vi "sk-watertunnel-control-9-10-16.vi"() -> ()   [LabVIEW 2012]
uses:
  <vilib>/Utility/error.llb/DialogType.ctl
  <vilib>/DAQmx/write.llb/DAQmx Write (Digital 1D Wfm NChan NSamp).vi
  <vilib>/DAQmx/write.llb/DAQmx Write (Analog Wfm 1Chan NSamp).vi
  <vilib>/DAQmx/write.llb/DAQmx Write (Analog DBL 1Chan 1Samp).vi
  <vilib>/DAQmx/write.llb/DAQmx Write (Digital 1D Bool 1Chan 1Samp).vi
  <vilib>/Instr/_visa.llb/VISA Configure Serial Port (Instr).vi
  <vilib>/DAQmx/create/channels.llb/DAQmx Create Channel (AO-Voltage-Basic).vi
  <vilib>/DAQmx/create/channels.llb/DAQmx Create Channel (DO-Digital Output).vi
  <vilib>/Waveform/DWDTOps.llb/DWDT Analog to Digital.vi
  <vilib>/DAQmx/configure/timing.llb/DAQmx Timing (Sample Clock).vi
  <vilib>/DAQmx/create/channels.llb/DAQmx Create Channel (CO-Pulse Generation-Time).vi
  <vilib>/DAQmx/configure/trigger.llb/DAQmx Start Trigger (Digital Edge).vi
  <vilib>/DAQmx/miscellaneous.llb/DAQmx Fill In Error Info.vi
  <vilib>/Waveform/DWDTOps.llb/DWDT Uncompress Digital.vi
  <vilib>/measure/NI_MABase.lvlib
panel:
  in  "RECORD":bool
  in  "select path":path=path "D:/skramel/labview/hex-9-6-2016-2-15-1-01.txt"
  in  "VISA resource name 5":refnum<visa-resource-name>="COM105"
  in  "VISA resource name 4":refnum<visa-resource-name>="COM104"
  in  "VISA resource name 3":refnum<visa-resource-name>="COM103"
  in  "VISA resource name 2":refnum<visa-resource-name>="COM102"
  in  "Select Program":i32(ring)=1 items=["Manual Control", "Read from .txt file"]
  in  "stop":bool
  out "Current Command in .txt file - board 1":string="relay writeall 30\r"
  out "Current Command in .txt file - board 2":string="relay writeall 00\r"
  out "Current Command in .txt file - board 3":string="relay writeall 23\r"
  out "Current Command in .txt file - board 4":string="relay writeall 04\r"
  out "Current Command in .txt file - board 5":string="relay writeall 44\r"
  in  "Serial write":bool=TRUE
  in  "stop 2":bool
  in  "R 1":bool=TRUE
  in  "R 2":bool=TRUE
  in  "R 3":bool=TRUE
  in  "R 4":bool=TRUE
  in  "R 5":bool=TRUE
  in  "R 6":bool=TRUE
  in  "R 9":bool=TRUE
  in  "R 10":bool=TRUE
  in  "R 11":bool=TRUE
  in  "R 12":bool=TRUE
  in  "R 13":bool=TRUE
  in  "R 14":bool=TRUE
  in  "R 15":bool=TRUE
  in  "R 16":bool=TRUE
  in  "R 7":bool=TRUE
  in  "R 8":bool=TRUE
  in  "R 17":bool=TRUE
  in  "R 18":bool=TRUE
  in  "R 19":bool=TRUE
  in  "R 20":bool=TRUE
  in  "R 21":bool=TRUE
  in  "R 22":bool=TRUE
  in  "R 31":bool=TRUE
  in  "R 32":bool=TRUE
  in  "R 23":bool=TRUE
  in  "R 24":bool=TRUE
  in  "R 25":bool=TRUE
  in  "R 26":bool=TRUE
  in  "R 27":bool=TRUE
  in  "R 28":bool=TRUE
  in  "R 29":bool=TRUE
  in  "R 30":bool=TRUE
  out "Current Command (manual control) - board 1":string="relay writeall 00\r"
  in  "R 33":bool=TRUE
  in  "R 34":bool=TRUE
  in  "R 35":bool=TRUE
  in  "R 36":bool=TRUE
  in  "R 37":bool=TRUE
  in  "R 38":bool=TRUE
  in  "R 39":bool=TRUE
  in  "R 40":bool=TRUE
  out "Current Command (manual control) - board 2":string="relay writeall 00\r"
  out "board 5":string="00"
  in  "Manual Override - turn all relays off":bool=TRUE
  out "board 1":string="00"
  out "board 2":string="00"
  out "board 3":string="00"
  out "board 4":string="00"
  out "Current Command (manual control) - board 3":string="relay writeall 00\r"
  out "Current Command (manual control) - board 4":string="relay writeall 00\r"
  out "Current Command (manual control) - board 5":string="relay writeall 00\r"
  in  "Serial write update rate (ms)":u32=100
  in  "End write with termination character?":bool=TRUE
  in  "Input buffer size":u32=4096
  in  "termination char\n(0xA = '\\n' = LF\n0xD = '\\r' = CR)":u8=13 format="%.0x"
  in  "End read on termination character?":bool=TRUE
  in  "timeout (ms)":u32=10000
  in  "stop bits":u16(ring)=10 items=["1.0"=10, "1.5"=15, "2.0"=20]
  in  "parity":u16(ring) items=["None", "Odd", "Even", "Mark", "Space"]
  in  "data bits":u16=8 min=5 max=8 step=1
  in  "VISA resource name 1":refnum<visa-resource-name>="COM101"
  in  "baud rate":u32=9600
  in  "Physical Channel":tag="Dev1/ao1" caption="Analog Output (LED Trigger - Black Wire)"
  in  "duty cycle (%)":dbl=10.0 format="%0.2f"
  in  "phase":dbl format="%.2p"
  in  "amplitude":dbl=10.0 format="%0.2p"
  in  "frequency":dbl=450.0 format="%0.2p"
  in  "STOP":bool
  in  "sampling info":cluster{"Fs":dbl, "#s":dbl}={"Fs"=450000.0, "#s"=450000.0} {"Fs" format="%.2p"}
  in  "duty cycle (%)":dbl=50.0 format="%0.2f"
  in  "phase":dbl format="%.2p"
  in  "amplitude":dbl=1.0 format="%0.2p"
  in  "frequency":dbl=450.0 format="%0.2p"
  in  "Sample Clock Rate":dbl=450000.0 format="%.2f"
  in  "Digital Output (Camera Trigger)":tag="Dev1/port0/line0:1" caption="Physical Channels"
  in  "On / Off":bool=TRUE
  in  "Voltage Output":dbl(slide)=10.0 min=0.0 max=10.0 scale=0.0..10.0 scale format="%.3f"
  in  "Maximum Value":dbl=10.0 format="%0.2f"
  in  "Minimum Value":dbl format="%0.2f"
  in  "Physical Channel":tag="Dev1/ao0" caption="Analog Output (LED Intensity - Grey Wire)"
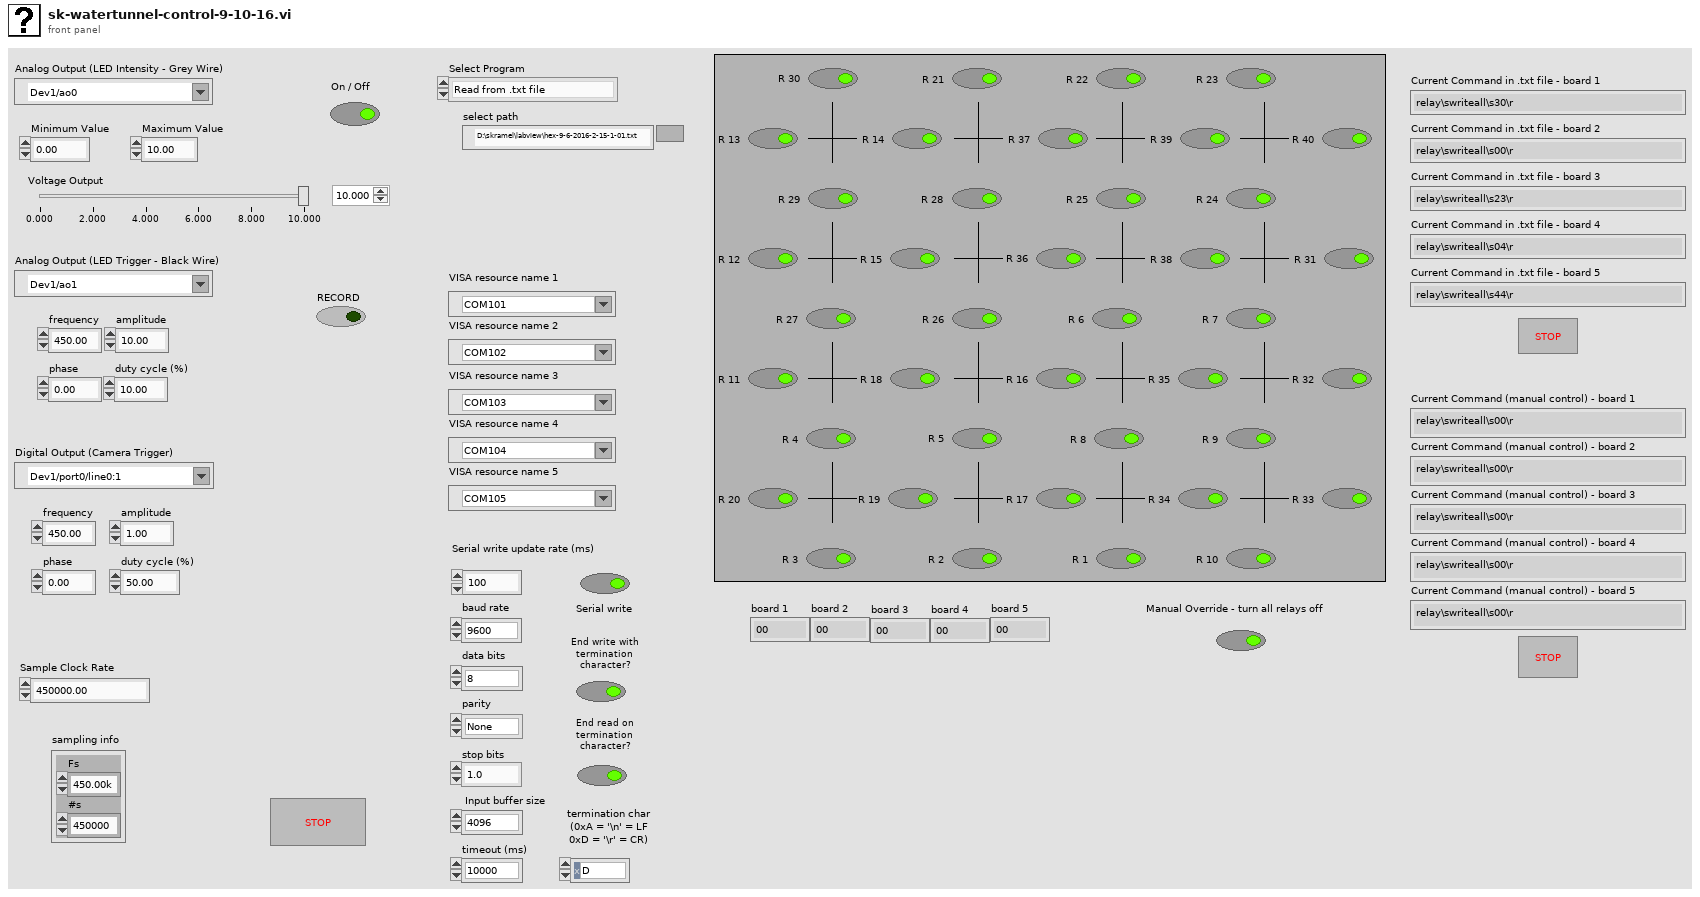
[diagram p1: front panel]
types:
  T1 = enum16{"open", "replace", "create", "open or create", "replace or create", "replace or create with confirmation"}
  T2 = typedef "DialogType.ctl" = u16
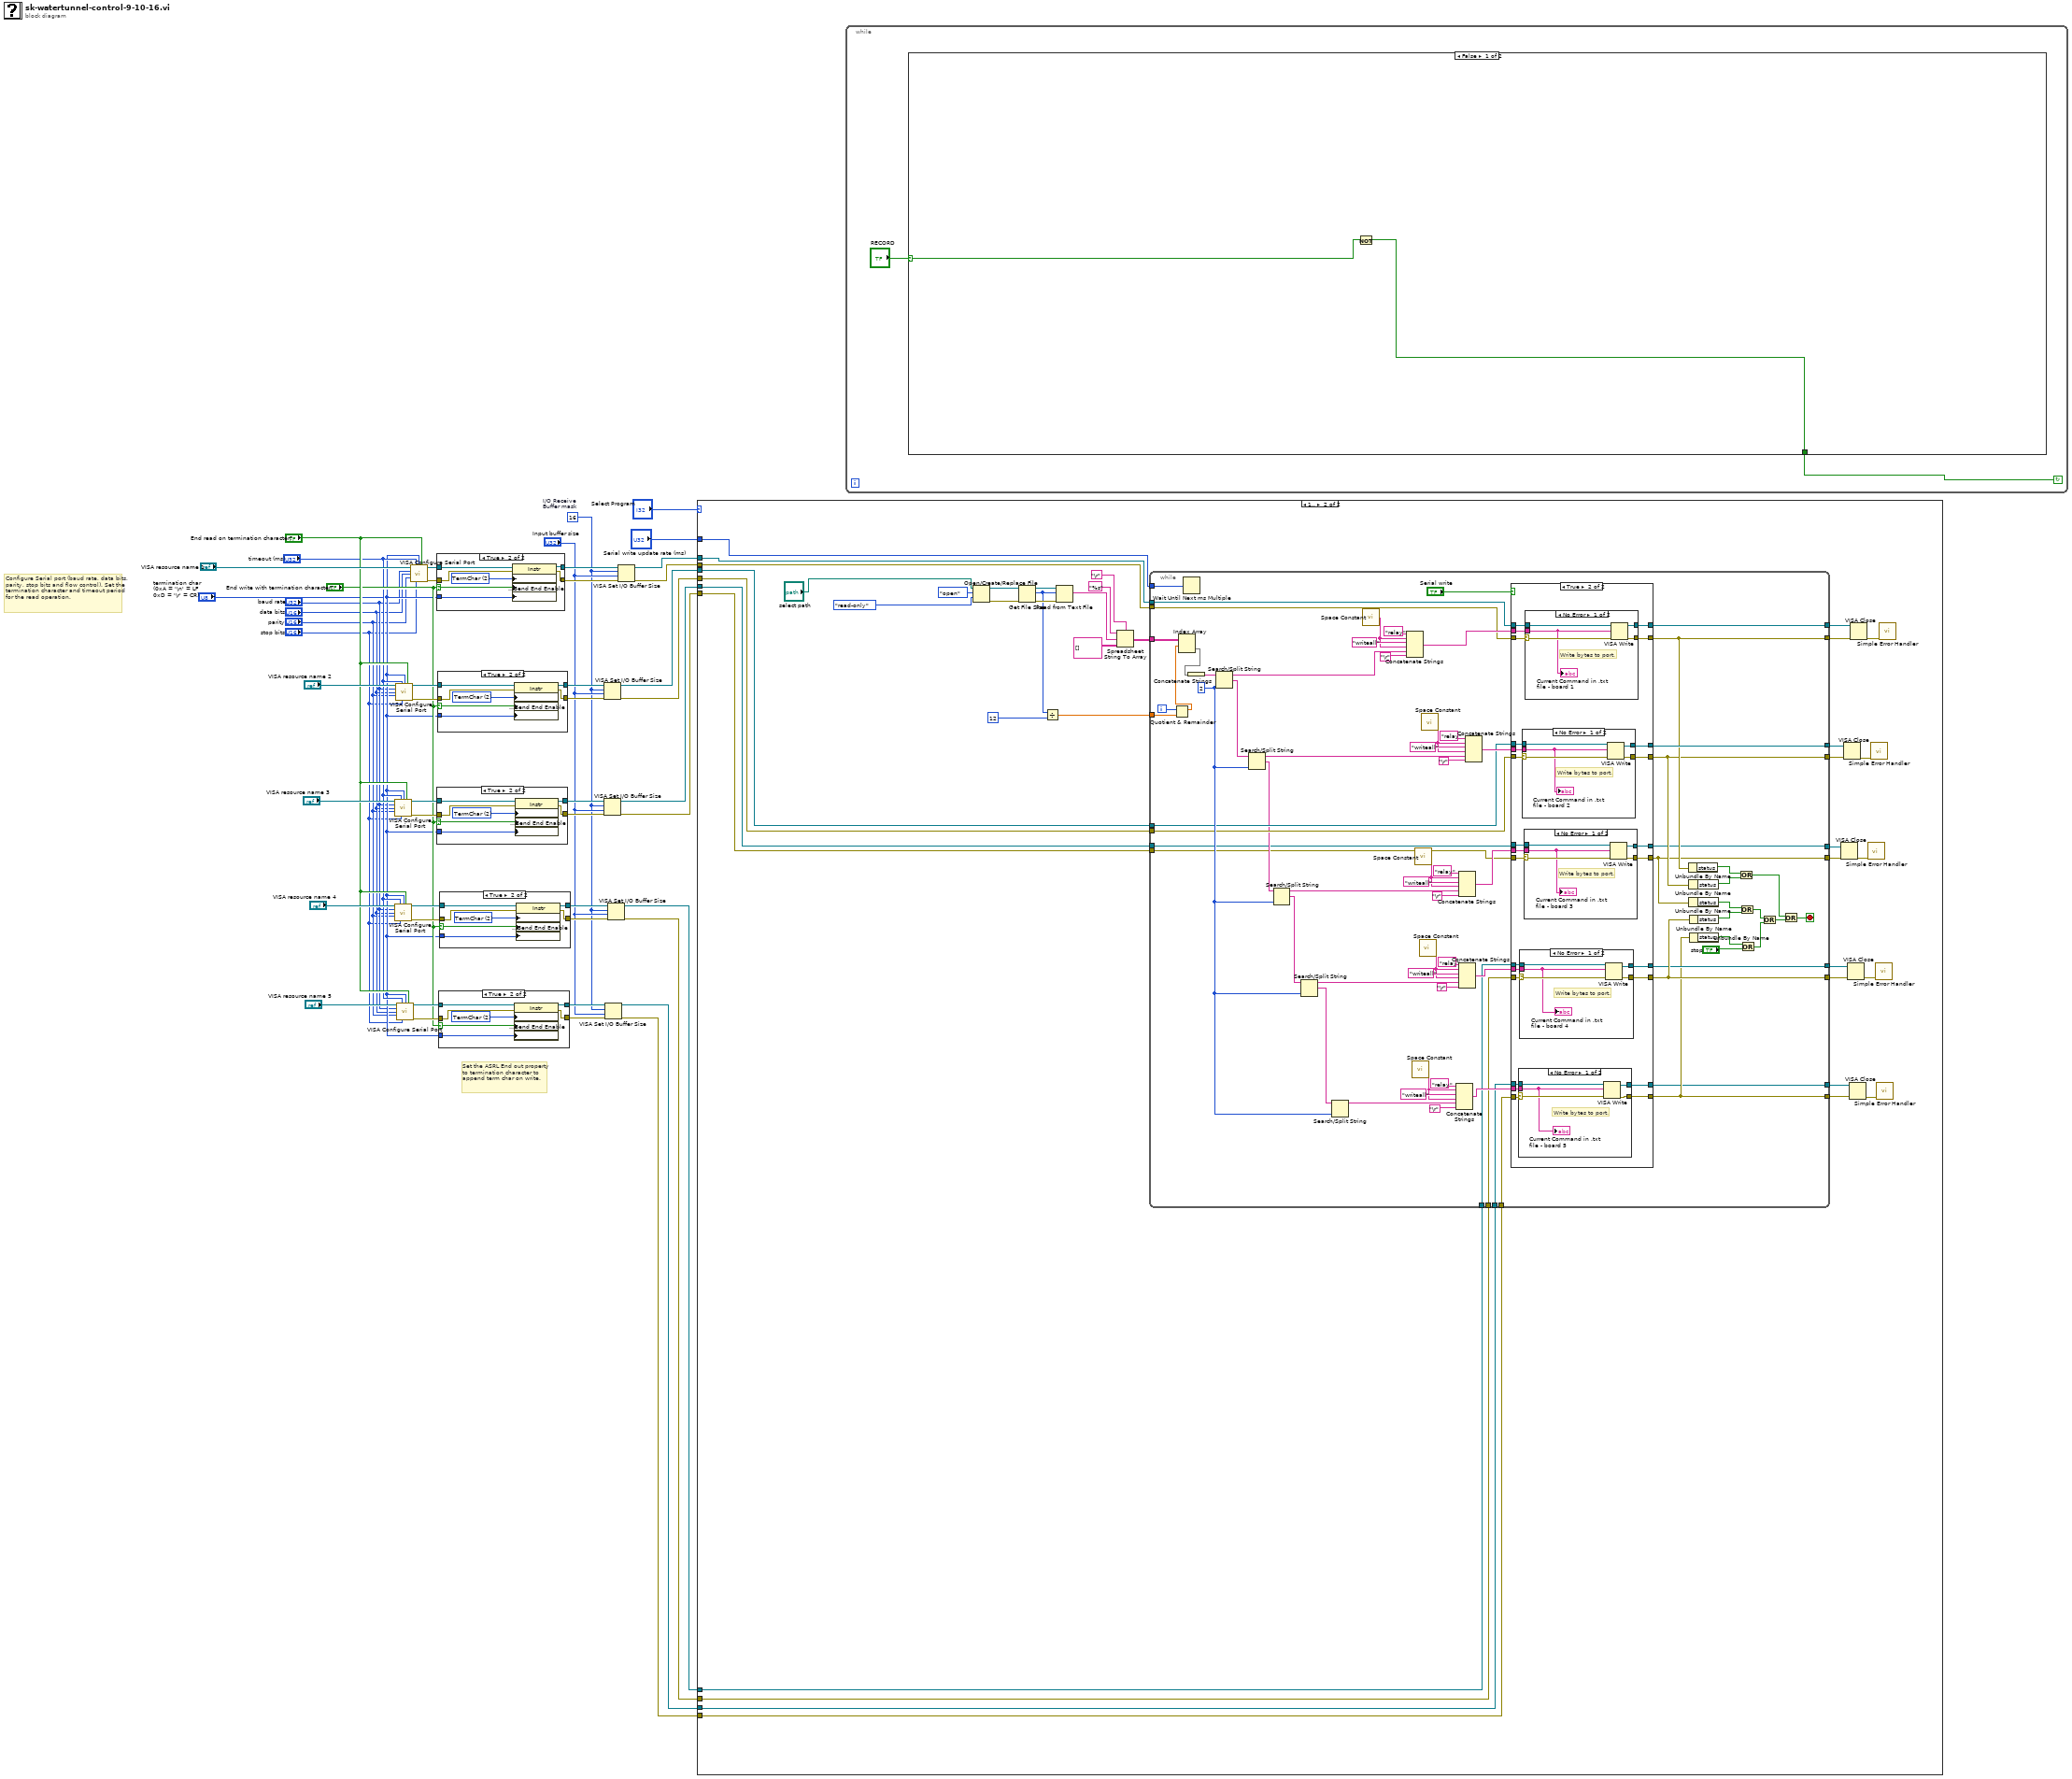
[diagram p0: block diagram]
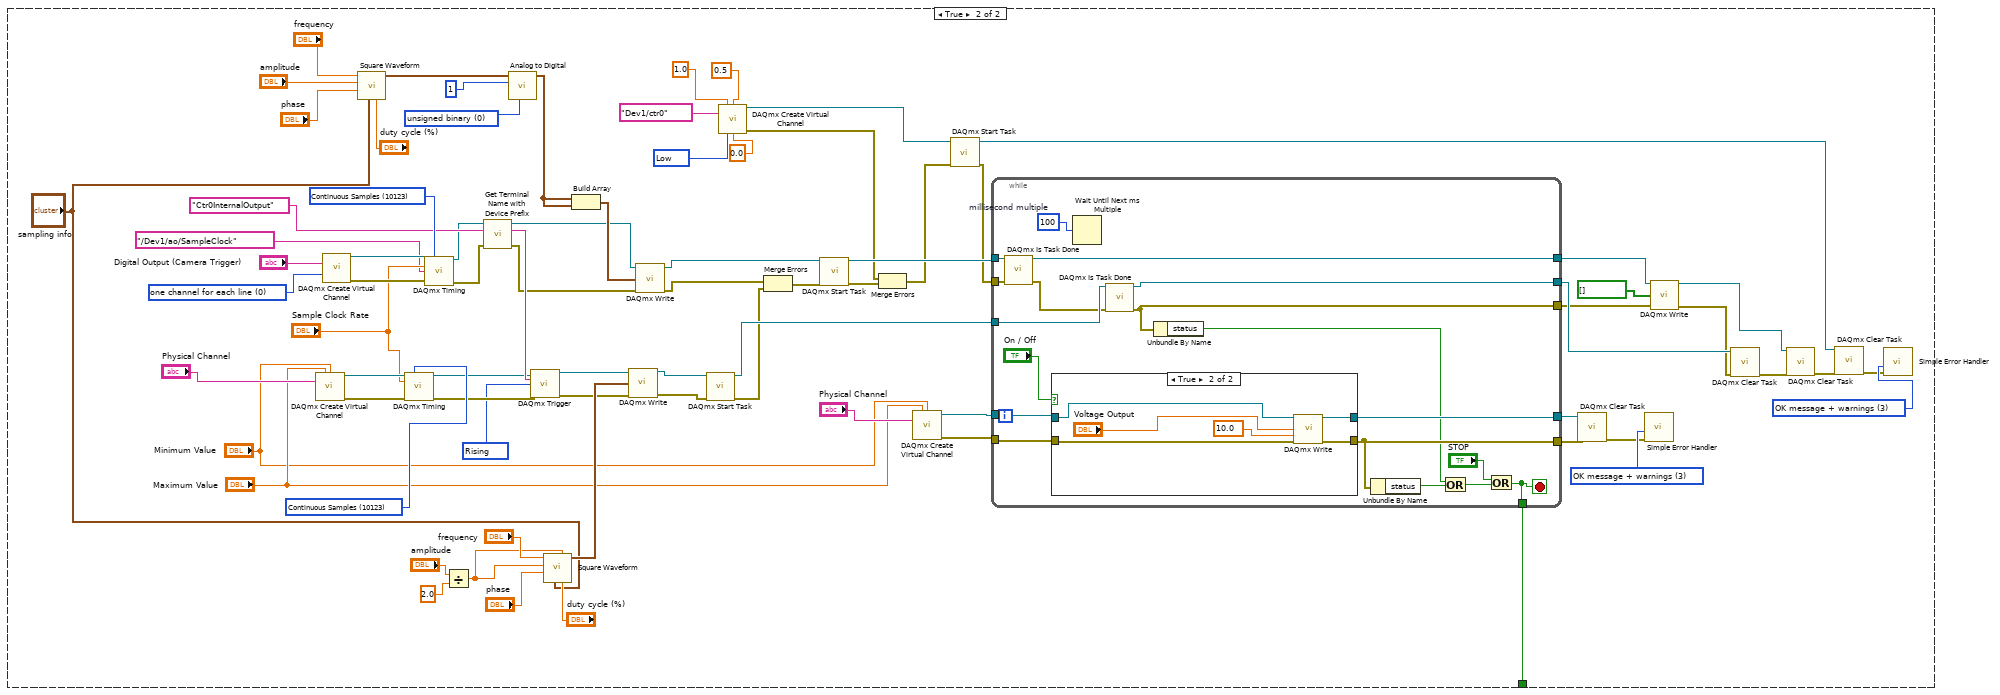
[diagram p2: hidden frame]
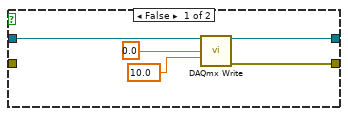
[diagram p3: hidden frame]
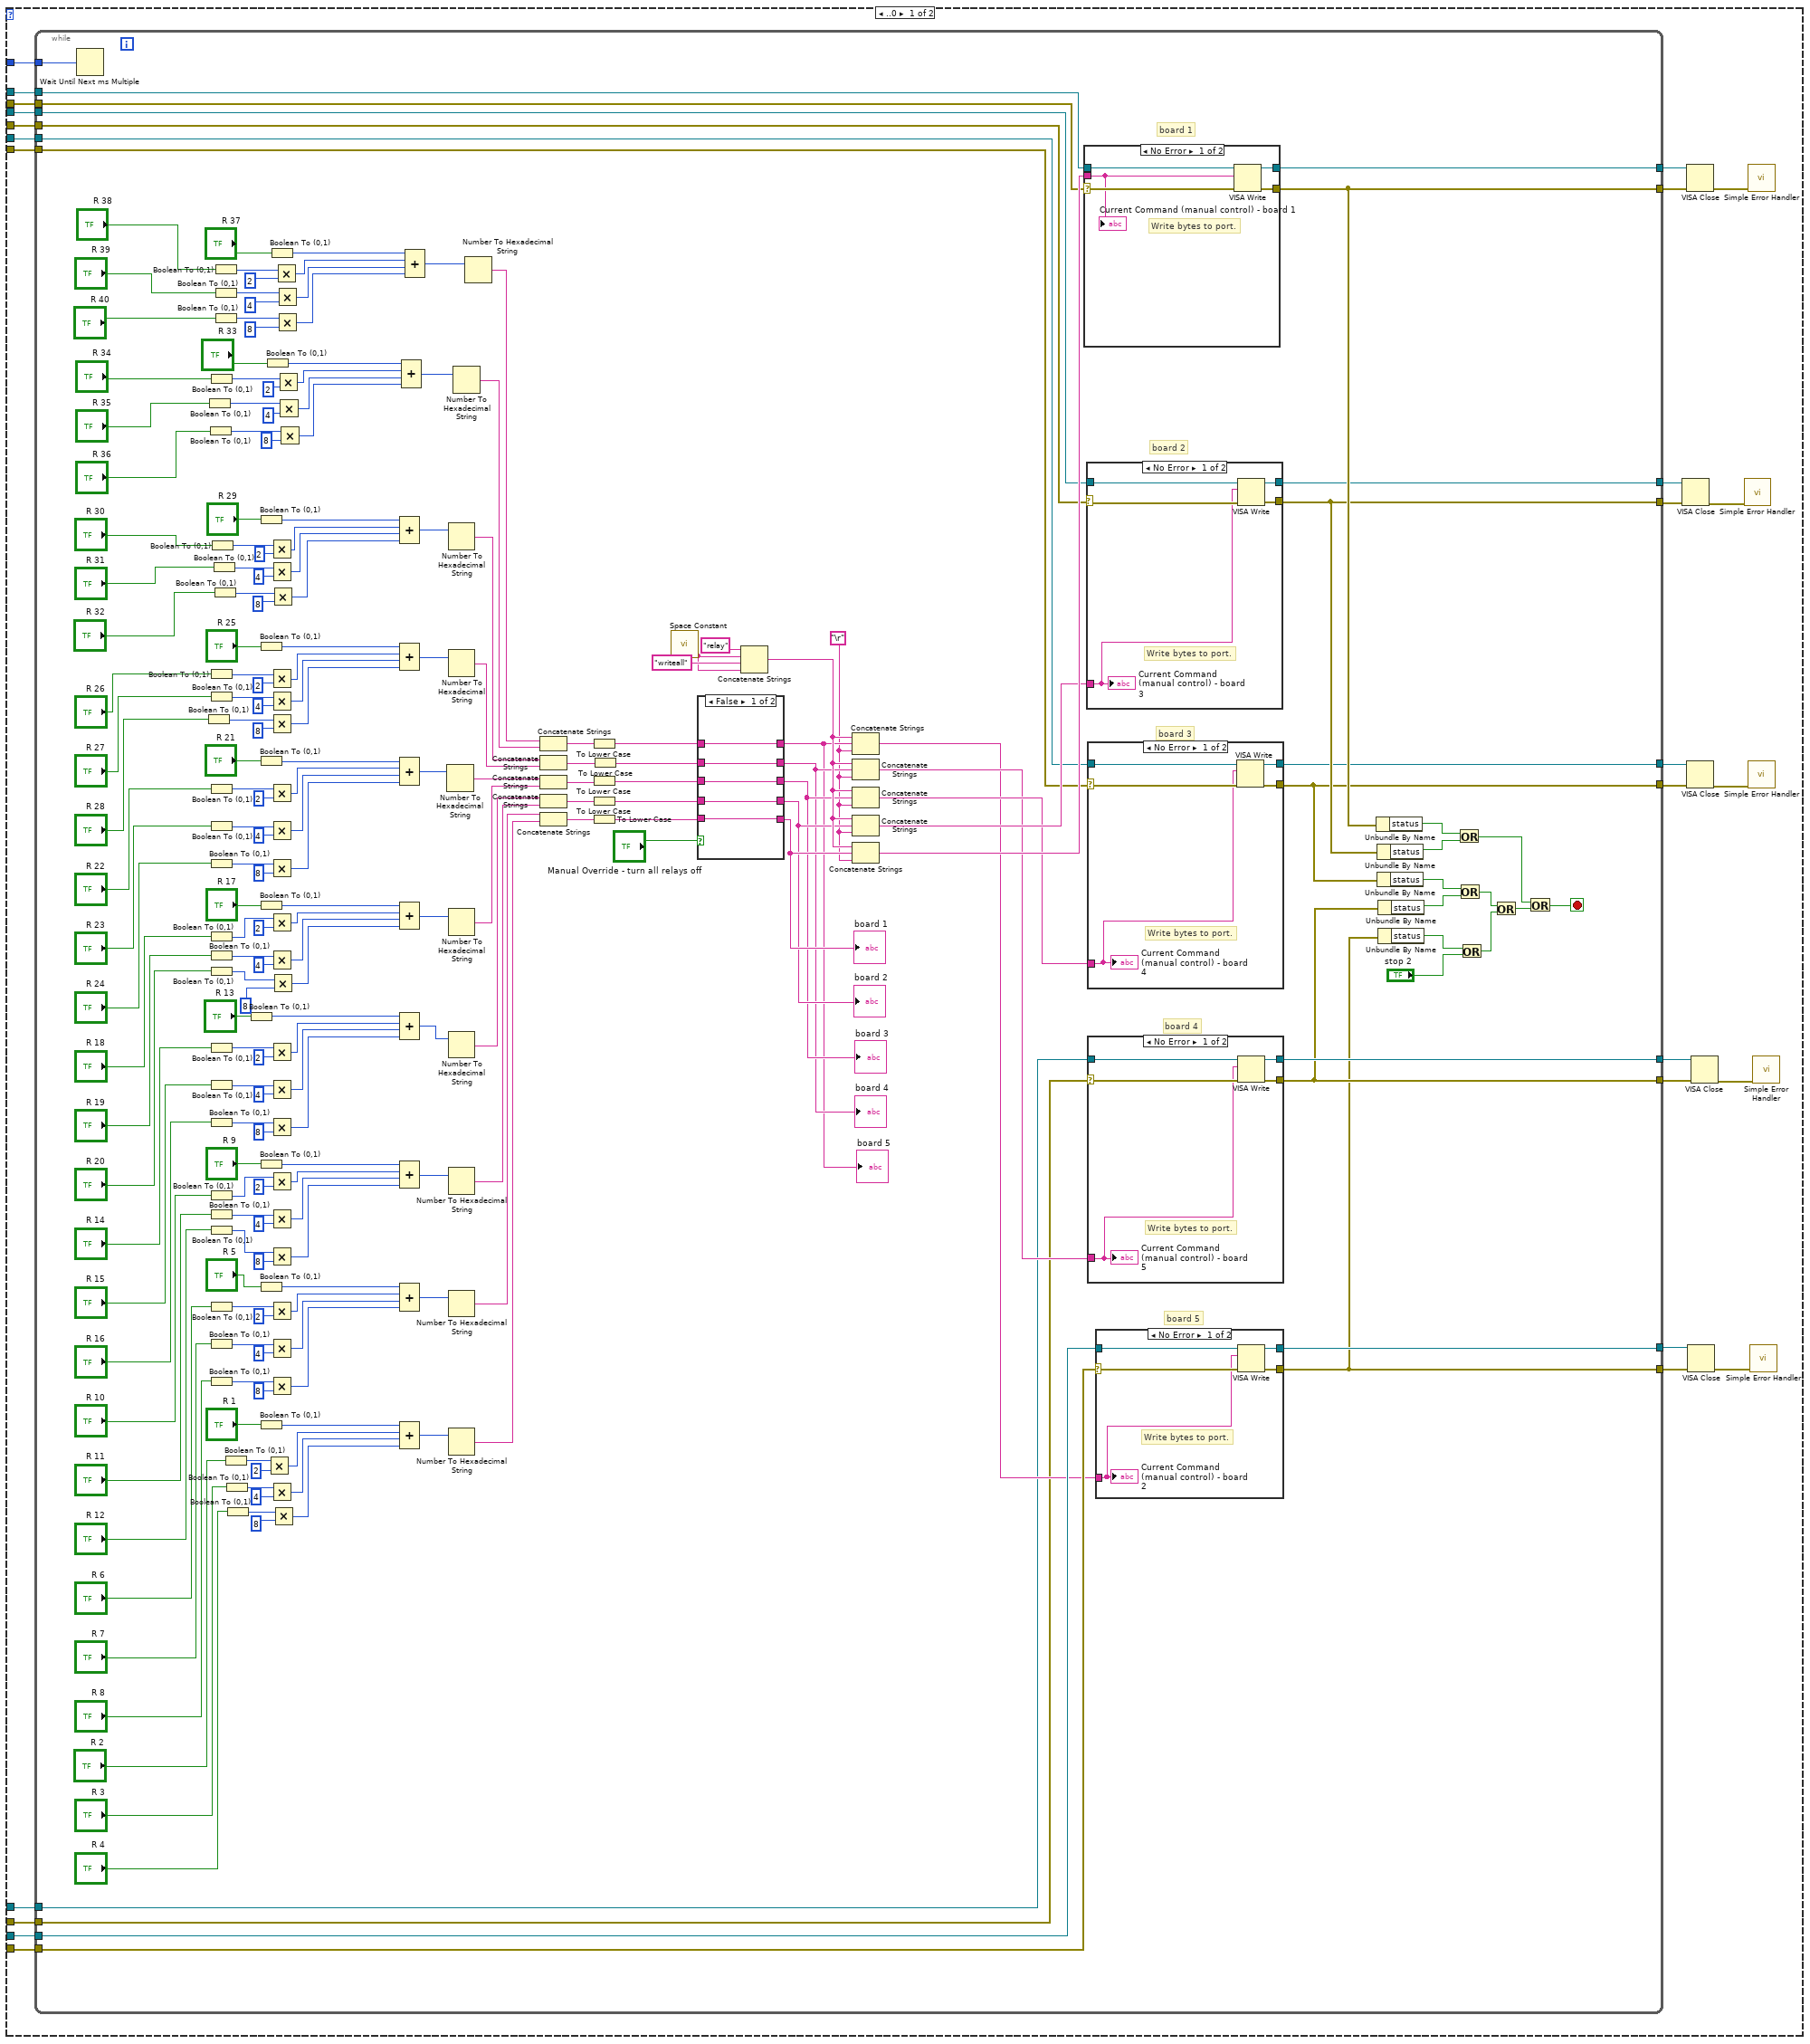
[diagram p8: hidden frame]
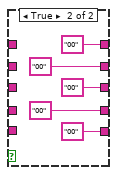
[diagram p12: hidden frame]
diagram:
  w1 = u16 16  # I/O Receive Buffer mask
  # "Set the ASRL End out property to termination character to append term char on write."
  # "Configure Serial port (baud rate, data bits, parity, stop bits and flow control). Set the termination character and timeout period for the read operation."
  n1 = call-poly "VISA Configure Serial Port"("VISA resource name"="VISA resource name 4", "timeout (10sec)"="timeout (ms)", "termination char\n(0xA = '\\n' = LF)"="termination char\n(0xA = '\\n' = LF\n0xD = '\\r' = CR)", "Enable Termination\nChar (T)"="End read on termination character?", "baud rate (9600)"="baud rate", "data bits (8)"="data bits", "parity (0:none)"="parity", "stop bits (10: 1 bit)"="stop bits") -> ("VISA resource name out"=w23:refnum<visa-resource-name>, "error out"=w26:errorcluster)  [unwired: 2 in, 4 out]
  n2 = call-poly "VISA Configure Serial Port"("VISA resource name"="VISA resource name 3", "timeout (10sec)"="timeout (ms)", "termination char\n(0xA = '\\n' = LF)"="termination char\n(0xA = '\\n' = LF\n0xD = '\\r' = CR)", "Enable Termination\nChar (T)"="End read on termination character?", "baud rate (9600)"="baud rate", "data bits (8)"="data bits", "parity (0:none)"="parity", "stop bits (10: 1 bit)"="stop bits") -> ("VISA resource name out"=w28:refnum<visa-resource-name>, "error out"=w31:errorcluster)  [unwired: 2 in, 4 out]
  n3 = call-poly "VISA Configure Serial Port"("VISA resource name"="VISA resource name 2", "timeout (10sec)"="timeout (ms)", "termination char\n(0xA = '\\n' = LF)"="termination char\n(0xA = '\\n' = LF\n0xD = '\\r' = CR)", "Enable Termination\nChar (T)"="End read on termination character?", "baud rate (9600)"="baud rate", "data bits (8)"="data bits", "parity (0:none)"="parity", "stop bits (10: 1 bit)"="stop bits") -> ("VISA resource name out"=w35:refnum<visa-resource-name>, "error out"=w38:errorcluster)  [unwired: 2 in, 4 out]
  n4 = call-poly "VISA Configure Serial Port"("VISA resource name"="VISA resource name 5", "timeout (10sec)"="timeout (ms)", "termination char\n(0xA = '\\n' = LF)"="termination char\n(0xA = '\\n' = LF\n0xD = '\\r' = CR)", "Enable Termination\nChar (T)"="End read on termination character?", "baud rate (9600)"="baud rate", "data bits (8)"="data bits", "parity (0:none)"="parity", "stop bits (10: 1 bit)"="stop bits") -> ("VISA resource name out"=w18:refnum<visa-resource-name>, "error out"=w21:errorcluster)  [unwired: 2 in, 4 out]
  n5 = call-poly "VISA Configure Serial Port"("VISA resource name"="VISA resource name 1", "timeout (10sec)"="timeout (ms)", "termination char\n(0xA = '\\n' = LF)"="termination char\n(0xA = '\\n' = LF\n0xD = '\\r' = CR)", "Enable Termination\nChar (T)"="End read on termination character?", "baud rate (9600)"="baud rate", "data bits (8)"="data bits", "parity (0:none)"="parity", "stop bits (10: 1 bit)"="stop bits") -> ("VISA resource name out"=w43:refnum<visa-resource-name>, "error out"=w46:errorcluster)  [unwired: 2 in, 4 out]
  n6 = case shown="True" "End write with termination character?" {
    selector: "End write with termination character?" -> [_ w51]
    tunnel: w43 -> [w48 w56]
    tunnel: w46 -> [w49 w55]
    tunnel: [w48 w54] -> w44
    tunnel: [w49 w50] -> w45
    tunnel: "termination char\n(0xA = '\\n' = LF\n0xD = '\\r' = CR)" -> [_ w52]
    frame False {
    }
    frame True {
      w53 = u16 2 items=["None", "LastBit", "TermChar", "Break"] ("Serial Settings:Serial End Mode for Writes")
      n7 = property class="Instr"(reference=w56, error in=w55, "Serial Settings:End Mode for Writes"=w53, "Message Based Settings:Send End Enable"=w51, "Message Based Settings:Termination Character"=w52) -> (reference out=w54:refnum<visa-resource-name>, error out=w50:errorcluster)
    }
  }
  n8 = case shown="True" "End write with termination character?" {
    selector: "End write with termination character?" -> [_ w60]
    tunnel: w28 -> [w57 w65]
    tunnel: w31 -> [w58 w64]
    tunnel: [w57 w63] -> w29
    tunnel: [w58 w62] -> w30
    tunnel: "termination char\n(0xA = '\\n' = LF\n0xD = '\\r' = CR)" -> [_ w59]
    frame False {
    }
    frame True {
      w61 = u16 2 items=["None", "LastBit", "TermChar", "Break"] ("Serial Settings:Serial End Mode for Writes")
      n9 = property class="Instr"(reference=w65, error in=w64, "Serial Settings:End Mode for Writes"=w61, "Message Based Settings:Send End Enable"=w60, "Message Based Settings:Termination Character"=w59) -> (reference out=w63:refnum<visa-resource-name>, error out=w62:errorcluster)
    }
  }
  n10 = case shown="True" "End write with termination character?" {
    selector: "End write with termination character?" -> [_ w69]
    tunnel: w35 -> [w66 w74]
    tunnel: w38 -> [w67 w73]
    tunnel: [w66 w72] -> w36
    tunnel: [w67 w71] -> w37
    tunnel: "termination char\n(0xA = '\\n' = LF\n0xD = '\\r' = CR)" -> [_ w68]
    frame False {
    }
    frame True {
      w70 = u16 2 items=["None", "LastBit", "TermChar", "Break"] ("Serial Settings:Serial End Mode for Writes")
      n11 = property class="Instr"(reference=w74, error in=w73, "Serial Settings:End Mode for Writes"=w70, "Message Based Settings:Send End Enable"=w69, "Message Based Settings:Termination Character"=w68) -> (reference out=w72:refnum<visa-resource-name>, error out=w71:errorcluster)
    }
  }
  n12 = case shown="True" "End write with termination character?" {
    selector: "End write with termination character?" -> [_ w78]
    tunnel: w18 -> [w75 w83]
    tunnel: w21 -> [w76 w82]
    tunnel: [w75 w81] -> w19
    tunnel: [w76 w80] -> w20
    tunnel: "termination char\n(0xA = '\\n' = LF\n0xD = '\\r' = CR)" -> [_ w77]
    frame False {
    }
    frame True {
      w79 = u16 2 items=["None", "LastBit", "TermChar", "Break"] ("Serial Settings:Serial End Mode for Writes")
      n13 = property class="Instr"(reference=w83, error in=w82, "Serial Settings:End Mode for Writes"=w79, "Message Based Settings:Send End Enable"=w78, "Message Based Settings:Termination Character"=w77) -> (reference out=w81:refnum<visa-resource-name>, error out=w80:errorcluster)
    }
  }
  n14 = case shown="True" "End write with termination character?" {
    selector: "End write with termination character?" -> [_ w87]
    tunnel: w23 -> [w84 w92]
    tunnel: w26 -> [w85 w91]
    tunnel: [w84 w90] -> w24
    tunnel: [w85 w89] -> w25
    tunnel: "termination char\n(0xA = '\\n' = LF\n0xD = '\\r' = CR)" -> [_ w86]
    frame False {
    }
    frame True {
      w88 = u16 2 items=["None", "LastBit", "TermChar", "Break"] ("Serial Settings:Serial End Mode for Writes")
      n15 = property class="Instr"(reference=w92, error in=w91, "Serial Settings:End Mode for Writes"=w88, "Message Based Settings:Send End Enable"=w87, "Message Based Settings:Termination Character"=w86) -> (reference out=w90:refnum<visa-resource-name>, error out=w89:errorcluster)
    }
  }
  n16 = VISA Set I/O Buffer Size(VISA resource name=w29, mask (16)=w1, size (4096)="Input buffer size", error in (no error)=w30) -> (VISA resource name out=w8:refnum<visa-resource-name>, error out=w7:errorcluster)
  n17 = VISA Set I/O Buffer Size(VISA resource name=w36, mask (16)=w1, size (4096)="Input buffer size", error in (no error)=w37) -> (VISA resource name out=w34:refnum<visa-resource-name>, error out=w33:errorcluster)
  n18 = VISA Set I/O Buffer Size(VISA resource name=w19, mask (16)=w1, size (4096)="Input buffer size", error in (no error)=w20) -> (VISA resource name out=w5:refnum<visa-resource-name>, error out=w6:errorcluster)
  n19 = VISA Set I/O Buffer Size(VISA resource name=w24, mask (16)=w1, size (4096)="Input buffer size", error in (no error)=w25) -> (VISA resource name out=w3:refnum<visa-resource-name>, error out=w4:errorcluster)
  n20 = VISA Set I/O Buffer Size(VISA resource name=w44, mask (16)=w1, size (4096)="Input buffer size", error in (no error)=w45) -> (VISA resource name out=w42:refnum<visa-resource-name>, error out=w41:errorcluster)
  n21 = case shown="1.." "Select Program" {
    tunnel: w42 -> [w114 w410]
    tunnel: w41 -> [w110 w409]
    tunnel: "Serial write update rate (ms)" -> [w115 w408]
    tunnel: w34 -> [w109 w407]
    tunnel: w33 -> [w108 w406]
    tunnel: w8 -> [w107 w384]
    tunnel: w7 -> [w106 w383]
    tunnel: w6 -> [w105 w385]
    tunnel: w5 -> [w104 w386]
    tunnel: w4 -> [w103 w387]
    tunnel: w3 -> [w102 w388]
    frame ..0 {
      n22 = while {
        tunnel: w114 -> [w335]
        tunnel: [w334] -> w117
        tunnel: [w143] -> w116
        tunnel: w115 -> [w333]
        tunnel: w104 -> [w150]
        tunnel: w105 -> [w212]
        tunnel: [w211] -> w112
        tunnel: [w139] -> w98
        tunnel: [w140] -> w97
        tunnel: [w137] -> w96
        tunnel: [w138] -> w95
        tunnel: [w136] -> w93
        tunnel: [w135] -> w94
        tunnel: [w134] -> w111
        tunnel: w110 -> [w124]
        tunnel: w109 -> [w125]
        tunnel: w108 -> [w126]
        tunnel: w107 -> [w123]
        tunnel: w106 -> [w122]
        tunnel: w103 -> [w121]
        tunnel: w102 -> [w120]
        stop <- w127 stop-if-true
        w119 = "\r"
        # "board 2"
        # "board 5"
        # "board 4"
        # "board 3"
        # "board 1"
        n23 = Wait Until Next ms Multiple(millisecond multiple=w333) -> ()  [unwired: 1 out]
        n24 = Boolean To (0,1)(Boolean="R 28") -> (0, 1=w242:i16)
        n25 = Boolean To (0,1)(Boolean="R 35") -> (0, 1=w190:i16)
        n26 = Boolean To (0,1)(Boolean="R 36") -> (0, 1=w188:i16)
        n27 = Boolean To (0,1)(Boolean="R 34") -> (0, 1=w192:i16)
        n28 = Boolean To (0,1)(Boolean="R 26") -> (0, 1=w246:i16)
        n29 = Boolean To (0,1)(Boolean="R 27") -> (0, 1=w244:i16)
        n30 = Boolean To (0,1)(Boolean="R 22") -> (0, 1=w257:i16)
        n31 = Boolean To (0,1)(Boolean="R 23") -> (0, 1=w255:i16)
        n32 = Boolean To (0,1)(Boolean="R 24") -> (0, 1=w253:i16)
        n33 = Boolean To (0,1)(Boolean="R 18") -> (0, 1=w268:i16)
        n34 = Boolean To (0,1)(Boolean="R 19") -> (0, 1=w266:i16)
        n35 = Boolean To (0,1)(Boolean="R 20") -> (0, 1=w264:i16)
        n36 = Boolean To (0,1)(Boolean="R 14") -> (0, 1=w295:i16)
        n37 = Boolean To (0,1)(Boolean="R 15") -> (0, 1=w293:i16)
        n38 = Boolean To (0,1)(Boolean="R 16") -> (0, 1=w291:i16)
        n39 = Boolean To (0,1)(Boolean="R 10") -> (0, 1=w306:i16)
        n40 = Boolean To (0,1)(Boolean="R 11") -> (0, 1=w304:i16)
        n41 = Boolean To (0,1)(Boolean="R 12") -> (0, 1=w302:i16)
        n42 = Boolean To (0,1)(Boolean="R 6") -> (0, 1=w317:i16)
        n43 = Boolean To (0,1)(Boolean="R 7") -> (0, 1=w315:i16)
        n44 = Boolean To (0,1)(Boolean="R 8") -> (0, 1=w313:i16)
        n45 = Boolean To (0,1)(Boolean="R 30") -> (0, 1=w235:i16)
        n46 = Boolean To (0,1)(Boolean="R 31") -> (0, 1=w233:i16)
        n47 = Boolean To (0,1)(Boolean="R 32") -> (0, 1=w231:i16)
        n48 = Boolean To (0,1)(Boolean="R 38") -> (0, 1=w181:i16)
        n49 = Boolean To (0,1)(Boolean="R 39") -> (0, 1=w179:i16)
        n50 = Boolean To (0,1)(Boolean="R 40") -> (0, 1=w177:i16)
        n51 = Boolean To (0,1)(Boolean="R 2") -> (0, 1=w328:i16)
        n52 = Boolean To (0,1)(Boolean="R 3") -> (0, 1=w326:i16)
        n53 = Boolean To (0,1)(Boolean="R 4") -> (0, 1=w324:i16)
        n54 = Boolean To (0,1)(Boolean="R 13") -> (0, 1=w289:i16)
        n55 = Boolean To (0,1)(Boolean="R 29") -> (0, 1=w229:i16)
        n56 = Boolean To (0,1)(Boolean="R 25") -> (0, 1=w240:i16)
        n57 = Boolean To (0,1)(Boolean="R 21") -> (0, 1=w251:i16)
        n58 = Boolean To (0,1)(Boolean="R 17") -> (0, 1=w262:i16)
        n59 = Boolean To (0,1)(Boolean="R 9") -> (0, 1=w300:i16)
        n60 = Boolean To (0,1)(Boolean="R 5") -> (0, 1=w311:i16)
        n61 = Boolean To (0,1)(Boolean="R 1") -> (0, 1=w322:i16)
        n62 = Boolean To (0,1)(Boolean="R 33") -> (0, 1=w186:i16)
        n63 = Multiply(x=w328, y=i16 2) -> (x*y=w321:i16)
        n64 = Boolean To (0,1)(Boolean="R 37") -> (0, 1=w175:i16)
        n65 = Multiply(x=w235, y=i16 2) -> (x*y=w228:i16)
        n66 = Multiply(x=w233, y=i16 4) -> (x*y=w227:i16)
        n67 = Multiply(x=w246, y=i16 2) -> (x*y=w239:i16)
        n68 = Multiply(x=w244, y=i16 4) -> (x*y=w238:i16)
        n69 = Multiply(x=w242, y=i16 8) -> (x*y=w237:i16)
        n70 = Multiply(x=w257, y=i16 2) -> (x*y=w250:i16)
        n71 = Multiply(x=w255, y=i16 4) -> (x*y=w249:i16)
        n72 = Multiply(x=w253, y=i16 8) -> (x*y=w248:i16)
        n73 = Multiply(x=w268, y=i16 2) -> (x*y=w261:i16)
        n74 = Multiply(x=w266, y=i16 4) -> (x*y=w260:i16)
        n75 = Multiply(x=w295, y=i16 2) -> (x*y=w288:i16)
        n76 = Multiply(x=w293, y=i16 4) -> (x*y=w287:i16)
        n77 = Multiply(x=w291, y=i16 8) -> (x*y=w286:i16)
        n78 = Multiply(x=w306, y=i16 2) -> (x*y=w299:i16)
        n79 = Multiply(x=w304, y=i16 4) -> (x*y=w298:i16)
        n80 = Multiply(x=w302, y=i16 8) -> (x*y=w297:i16)
        n81 = Multiply(x=w317, y=i16 2) -> (x*y=w310:i16)
        n82 = Multiply(x=w315, y=i16 4) -> (x*y=w309:i16)
        n83 = Multiply(x=w313, y=i16 8) -> (x*y=w308:i16)
        n84 = Multiply(x=w326, y=i16 4) -> (x*y=w320:i16)
        n85 = Multiply(x=w231, y=i16 8) -> (x*y=w226:i16)
        n86 = Multiply(x=w264, y=i16 8) -> (x*y=w259:i16)
        n87 = Multiply(x=w324, y=i16 8) -> (x*y=w319:i16)
        n88 = Multiply(x=w181, y=i16 2) -> (x*y=w174:i16)
        n89 = Multiply(x=w179, y=i16 4) -> (x*y=w173:i16)
        n90 = Multiply(x=w177, y=i16 8) -> (x*y=w172:i16)
        n91 = Multiply(x=w192, y=i16 2) -> (x*y=w185:i16)
        n92 = Multiply(x=w190, y=i16 4) -> (x*y=w184:i16)
        n93 = Multiply(x=w188, y=i16 8) -> (x*y=w183:i16)
        n94 = Compound Arithmetic op=ADD(w229, w228, w227, w226) -> (w225:i16)
        n95 = Compound Arithmetic op=ADD(w240, w239, w238, w237) -> (w236:i16)
        n96 = Compound Arithmetic op=ADD(w251, w250, w249, w248) -> (w247:i16)
        n97 = Compound Arithmetic op=ADD(w262, w261, w260, w259) -> (w258:i16)
        n98 = Compound Arithmetic op=ADD(w289, w288, w287, w286) -> (w285:i16)
        n99 = Compound Arithmetic op=ADD(w300, w299, w298, w297) -> (w296:i16)
        n100 = Compound Arithmetic op=ADD(w311, w310, w309, w308) -> (w307:i16)
        n101 = Compound Arithmetic op=ADD(w322, w321, w320, w319) -> (w318:i16)
        n102 = Compound Arithmetic op=ADD(w186, w185, w184, w183) -> (w182:i16)
        n103 = Compound Arithmetic op=ADD(w175, w174, w173, w172) -> (w171:i16)
        n104 = Number To Hexadecimal String(2:w247) -> (0:w206:string)  [unwired: 1 in]
        n105 = Number To Hexadecimal String(2:w225) -> (0:w208:string)  [unwired: 1 in]
        n106 = Number To Hexadecimal String(2:w236) -> (0:w207:string)  [unwired: 1 in]
        n107 = Number To Hexadecimal String(2:w258) -> (0:w205:string)  [unwired: 1 in]
        n108 = Number To Hexadecimal String(2:w285) -> (0:w204:string)  [unwired: 1 in]
        n109 = Number To Hexadecimal String(2:w296) -> (0:w203:string)  [unwired: 1 in]
        n110 = Number To Hexadecimal String(2:w307) -> (0:w202:string)  [unwired: 1 in]
        n111 = Number To Hexadecimal String(2:w318) -> (0:w201:string)  [unwired: 1 in]
        n112 = Number To Hexadecimal String(2:w182) -> (0:w170:string)  [unwired: 1 in]
        n113 = Number To Hexadecimal String(2:w171) -> (0:w169:string)  [unwired: 1 in]
        n114 = Concatenate Strings(w169, w170) -> (w193:string)
        n115 = Concatenate Strings(w208, w207) -> (w199:string)
        n116 = Concatenate Strings(w206, w205) -> (w198:string)
        n117 = Concatenate Strings(w204, w203) -> (w197:string)
        n118 = Concatenate Strings(w202, w201) -> (w200:string)
        n119 = To Lower Case(string=w193) -> (all lower case string=w168:string)
        n120 = To Lower Case(string=w198) -> (all lower case string=w195:string)
        n121 = To Lower Case(string=w197) -> (all lower case string=w196:string)
        n122 = To Lower Case(string=w200) -> (all lower case string=w210:string)
        n123 = To Lower Case(string=w199) -> (all lower case string=w194:string)
        n124 = call <vilib>:"Space Constant.vi"() -> ("String"=w165:string)
        n125 = case shown="False" "Manual Override - turn all relays off" {
          tunnel: [w361 "00"] -> w154
          tunnel: w210 -> [w362 _]
          tunnel: [w359 "00"] -> w152
          tunnel: [w360 "00"] -> w153
          tunnel: [w362 "00"] -> w155
          tunnel: w196 -> [w361 _]
          tunnel: w195 -> [w360 _]
          tunnel: w194 -> [w359 _]
          tunnel: [w358 "00"] -> w151
          tunnel: w168 -> [w358 _]
          frame False {
          }
          frame True {
          }
        }
        "board 5" <- w151
        "board 1" <- w155
        "board 2" <- w154
        "board 3" <- w153
        "board 4" <- w152
        n126 = Concatenate Strings("relay", w165, "writeall", w165) -> (w164:string)
        n127 = Concatenate Strings(w164, w151, w119) -> (w145:string)
        n128 = Concatenate Strings(w164, w152, w119) -> (w146:string)
        n129 = Concatenate Strings(w164, w153, w119) -> (w147:string)
        n130 = Concatenate Strings(w164, w154, w119) -> (w148:string)
        n131 = Concatenate Strings(w164, w155, w119) -> (w149:string)
        n132 = case shown="No Error" w124 {
          selector: w124 -> [w376 w381]
          tunnel: [w379 w380] -> w334
          tunnel: [w378 w381] -> w143
          tunnel: w335 -> [w377 w380]
          tunnel: w149 -> [w375 _]
          frame No Error {
            # "Write bytes to port."
            n133 = VISA Write(VISA resource name=w377, write buffer=w375, error in (no error)=w376) -> (VISA resource name out=w379:refnum<visa-resource-name>, error out=w378:errorcluster)  [unwired: 1 out]
            "Current Command (manual control) - board 1" <- w375
          }
          frame Error {
          }
        }
        n134 = case shown="No Error" w126 {
          selector: w126 -> [w352 w357]
          tunnel: [w355 w356] -> w140
          tunnel: [w354 w357] -> w139
          tunnel: w125 -> [w353 w356]
          tunnel: w148 -> [w351 _]
          frame No Error {
            # "Write bytes to port."
            n135 = VISA Write(VISA resource name=w353, write buffer=w351, error in (no error)=w352) -> (VISA resource name out=w355:refnum<visa-resource-name>, error out=w354:errorcluster)  [unwired: 1 out]
            "Current Command (manual control) - board 3" <- w351
          }
          frame Error {
          }
        }
        n136 = case shown="No Error" w122 {
          selector: w122 -> [w346 w350]
          tunnel: [w348 w349] -> w138
          tunnel: [w347 w350] -> w137
          tunnel: w147 -> [w345 _]
          tunnel: w123 -> [w344 w349]
          frame No Error {
            # "Write bytes to port."
            n137 = VISA Write(VISA resource name=w344, write buffer=w345, error in (no error)=w346) -> (VISA resource name out=w348:refnum<visa-resource-name>, error out=w347:errorcluster)  [unwired: 1 out]
            "Current Command (manual control) - board 4" <- w345
          }
          frame Error {
          }
        }
        n138 = case shown="No Error" w121 {
          selector: w121 -> [w338 w343]
          tunnel: [w341 w342] -> w136
          tunnel: [w340 w343] -> w135
          tunnel: w120 -> [w339 w342]
          tunnel: w146 -> [w337 _]
          frame No Error {
            # "Write bytes to port."
            n139 = VISA Write(VISA resource name=w339, write buffer=w337, error in (no error)=w338) -> (VISA resource name out=w341:refnum<visa-resource-name>, error out=w340:errorcluster)  [unwired: 1 out]
            "Current Command (manual control) - board 5" <- w337
          }
          frame Error {
          }
        }
        n140 = case shown="No Error" w212 {
          selector: w212 -> [w369 w374]
          tunnel: [w372 w373] -> w211
          tunnel: [w371 w374] -> w134
          tunnel: w150 -> [w370 w373]
          tunnel: w145 -> [w368 _]
          frame No Error {
            # "Write bytes to port."
            n141 = VISA Write(VISA resource name=w370, write buffer=w368, error in (no error)=w369) -> (VISA resource name out=w372:refnum<visa-resource-name>, error out=w371:errorcluster)  [unwired: 1 out]
            "Current Command (manual control) - board 2" <- w368
          }
          frame Error {
          }
        }
        n142 = Unbundle By Name(w143) -> ("status"=w336:bool)
        n143 = Unbundle By Name(w139) -> ("status"=w144:bool)
        n144 = Unbundle By Name(w137) -> ("status"=w142:bool)
        n145 = Unbundle By Name(w135) -> ("status"=w141:bool)
        n146 = Unbundle By Name(w134) -> ("status"=w130:bool)
        n147 = Or(x=w336, y=w144) -> (x .or. y?=w132:bool)
        n148 = Or(x=w142, y=w141) -> (x .or. y?=w133:bool)
        n149 = Or(x=w130, y="stop 2") -> (x .or. y?=w128:bool)
        n150 = Or(x=w133, y=w128) -> (x .or. y?=w131:bool)
        n151 = Or(x=w132, y=w131) -> (x .or. y?=w127:bool)
      }
      n152 = VISA Close(VISA resource name=w97, error in (no error)=w98) -> (error out=w101:errorcluster)
      n153 = VISA Close(VISA resource name=w117, error in (no error)=w116) -> (error out=w118:errorcluster)
      n154 = VISA Close(VISA resource name=w95, error in (no error)=w96) -> (error out=w100:errorcluster)
      n155 = VISA Close(VISA resource name=w112, error in (no error)=w111) -> (error out=w113:errorcluster)
      n156 = VISA Close(VISA resource name=w93, error in (no error)=w94) -> (error out=w99:errorcluster)
      n157 = call <vilib>:"Simple Error Handler.vi"("error in (no error)"=w101) -> ()  [unwired: 1 in, 8 out]
      n158 = call <vilib>:"Simple Error Handler.vi"("error in (no error)"=w118) -> ()  [unwired: 1 in, 8 out]
      n159 = call <vilib>:"Simple Error Handler.vi"("error in (no error)"=w100) -> ()  [unwired: 1 in, 8 out]
      n160 = call <vilib>:"Simple Error Handler.vi"("error in (no error)"=w113) -> ()  [unwired: 1 in, 8 out]
      n161 = call <vilib>:"Simple Error Handler.vi"("error in (no error)"=w99) -> ()  [unwired: 1 in, 8 out]
    }
    frame 1.. {
      n162 = Open/Create/Replace File(file path (use dialog)="select path", operation (0:open)=T1."open", access (0:read/write)=enum16{"read/write", "read-only", "write-only"}."read-only") -> (refnum out=w419:refnum<file>, error out=w418:errorcluster)  [unwired: 1 in, 3 out]
      n163 = Get File Size(file=w419, error in=w418) -> (refnum out=w402:refnum<file>, size (in bytes)=w401:i64, 0:w403:errorcluster)
      n164 = Divide(x=w401, y=12) -> (x/y=w399:dbl)
      n165 = Read from Text File(file (use dialog)=w402, count=w401, error in=w403) -> (text=w416:string)  [unwired: 4 out]
      n166 = Spreadsheet String To Array(delimiter (Tab)="\r", format string="%s", spreadsheet string=w416, array type (2D Dbl)=string[][] [] ("Array")) -> (array=w411:string[][])
      n167 = while {
        tunnel: w410 -> [w496]
        tunnel: [w495] -> w413
        tunnel: [w438] -> w414
        tunnel: w409 -> [w489]
        tunnel: w411 -> [w479]
        tunnel: w408 -> [w488]
        tunnel: w407 -> [w453]
        tunnel: w406 -> [w454]
        tunnel: [w452] -> w398
        tunnel: [w437] -> w404
        tunnel: w399 -> [w478]
        tunnel: [w434] -> w394
        tunnel: [w433] -> w393
        tunnel: [w432] -> w391
        tunnel: [w431] -> w392
        tunnel: [w430] -> w390
        tunnel: [w429] -> w389
        tunnel: w388 -> [w425]
        tunnel: w387 -> [w426]
        tunnel: w386 -> [w427]
        tunnel: w385 -> [w428]
        tunnel: w384 -> [w424]
        tunnel: w383 -> [w423]
        i -> [w477]
        stop <- w439 stop-if-true
        w460 = 2
        n168 = Quotient & Remainder(x=w477, y=w478) -> (x-y*floor(x/y)=w476:dbl)  [unwired: 1 out]
        n169 = Index Array(array=w479, index (row)=w476) -> (element=w481:string[])  [unwired: 1 in]
        n170 = Wait Until Next ms Multiple(millisecond multiple=w488) -> ()  [unwired: 1 out]
        n171 = Concatenate Strings(w481) -> (w482:string)
        n172 = Search/Split String(string=w482, offset (0)=w460) -> (substring before match=w483:string, match + rest of string=w475:string)  [unwired: 1 in, 1 out]
        n173 = Search/Split String(string=w475, offset (0)=w460) -> (substring before match=w458:string, match + rest of string=w451:string)  [unwired: 1 in, 1 out]
        n174 = Search/Split String(string=w451, offset (0)=w460) -> (substring before match=w470:string, match + rest of string=w459:string)  [unwired: 1 in, 1 out]
        n175 = Search/Split String(string=w459, offset (0)=w460) -> (substring before match=w457:string, match + rest of string=w456:string)  [unwired: 1 in, 1 out]
        n176 = Search/Split String(string=w456, offset (0)=w460) -> (substring before match=w461:string)  [unwired: 1 in, 2 out]
        n177 = call <vilib>:"Space Constant.vi"() -> ("String"=w492:string)
        n178 = Concatenate Strings("relay", w492, "writeall", w492, w483, "\r") -> (w490:string)
        n179 = call <vilib>:"Space Constant.vi"() -> ("String"=w463:string)
        n180 = call <vilib>:"Space Constant.vi"() -> ("String"=w472:string)
        n181 = call <vilib>:"Space Constant.vi"() -> ("String"=w467:string)
        n182 = call <vilib>:"Space Constant.vi"() -> ("String"=w485:string)
        n183 = Concatenate Strings("relay", w463, "writeall", w463, w461, "\r") -> (w435:string)
        n184 = Concatenate Strings("relay", w472, "writeall", w472, w470, "\r") -> (w450:string)
        n185 = Concatenate Strings("relay", w467, "writeall", w467, w457, "\r") -> (w436:string)
        n186 = Concatenate Strings("relay", w485, "writeall", w485, w458, "\r") -> (w455:string)
        n187 = case shown="True" "Serial write" {
          tunnel: [w506 w531] -> w495
          tunnel: [w505 w530] -> w438
          tunnel: w496 -> [w506 w529]
          tunnel: w489 -> [w505 w528]
          tunnel: w490 -> [_ w527]
          tunnel: w455 -> [_ w524]
          tunnel: w454 -> [w503 w526]
          tunnel: w453 -> [w504 w525]
          tunnel: [w504 w523] -> w452
          tunnel: [w503 w522] -> w437
          tunnel: w450 -> [_ w521]
          tunnel: w424 -> [w502 w520]
          tunnel: w436 -> [_ w519]
          tunnel: w425 -> [w501 w518]
          tunnel: w435 -> [_ w517]
          tunnel: w427 -> [w500 w516]
          tunnel: [w498 w515] -> w432
          tunnel: [w497 w514] -> w430
          tunnel: [w499 w513] -> w434
          tunnel: [w502 w512] -> w433
          tunnel: [w501 w511] -> w431
          tunnel: [w500 w510] -> w429
          tunnel: w423 -> [w499 w507]
          tunnel: w426 -> [w498 w509]
          tunnel: w428 -> [w497 w508]
          frame False {
          }
          frame True {
            n188 = case shown="No Error" w508 {
              selector: w508 -> [w534 w538]
              tunnel: [w536 w537] -> w510
              tunnel: [w535 w538] -> w514
              tunnel: w517 -> [w532 _]
              tunnel: w516 -> [w533 w537]
              frame No Error {
                # "Write bytes to port."
                n189 = VISA Write(VISA resource name=w533, write buffer=w532, error in (no error)=w534) -> (VISA resource name out=w536:refnum<visa-resource-name>, error out=w535:errorcluster)  [unwired: 1 out]
                "Current Command in .txt file - board 5" <- w532
              }
              frame Error {
              }
            }
            n190 = case shown="No Error" w509 {
              selector: w509 -> [w541 w545]
              tunnel: [w543 w544] -> w511
              tunnel: [w542 w545] -> w515
              tunnel: w519 -> [w539 _]
              tunnel: w518 -> [w540 w544]
              frame No Error {
                # "Write bytes to port."
                n191 = VISA Write(VISA resource name=w540, write buffer=w539, error in (no error)=w541) -> (VISA resource name out=w543:refnum<visa-resource-name>, error out=w542:errorcluster)  [unwired: 1 out]
                "Current Command in .txt file - board 4" <- w539
              }
              frame Error {
              }
            }
            n192 = case shown="No Error" w526 {
              selector: w526 -> [w554 w559]
              tunnel: [w557 w558] -> w523
              tunnel: [w556 w559] -> w522
              tunnel: w525 -> [w555 w558]
              tunnel: w524 -> [w553 _]
              frame No Error {
                # "Write bytes to port."
                n193 = VISA Write(VISA resource name=w555, write buffer=w553, error in (no error)=w554) -> (VISA resource name out=w557:refnum<visa-resource-name>, error out=w556:errorcluster)  [unwired: 1 out]
                "Current Command in .txt file - board 2" <- w553
              }
              frame Error {
              }
            }
            n194 = case shown="No Error" w507 {
              selector: w507 -> [w548 w552]
              tunnel: [w550 w551] -> w512
              tunnel: [w549 w552] -> w513
              tunnel: w521 -> [w547 _]
              tunnel: w520 -> [w546 w551]
              frame No Error {
                # "Write bytes to port."
                n195 = VISA Write(VISA resource name=w546, write buffer=w547, error in (no error)=w548) -> (VISA resource name out=w550:refnum<visa-resource-name>, error out=w549:errorcluster)  [unwired: 1 out]
                "Current Command in .txt file - board 3" <- w547
              }
              frame Error {
              }
            }
            n196 = case shown="No Error" w528 {
              selector: w528 -> [w561 w566]
              tunnel: [w564 w565] -> w531
              tunnel: [w563 w566] -> w530
              tunnel: w529 -> [w562 w565]
              tunnel: w527 -> [w560 _]
              frame No Error {
                # "Write bytes to port."
                n197 = VISA Write(VISA resource name=w562, write buffer=w560, error in (no error)=w561) -> (VISA resource name out=w564:refnum<visa-resource-name>, error out=w563:errorcluster)  [unwired: 1 out]
                "Current Command in .txt file - board 1" <- w560
              }
              frame Error {
              }
            }
          }
        }
        n198 = Unbundle By Name(w438) -> ("status"=w449:bool)
        n199 = Unbundle By Name(w437) -> ("status"=w448:bool)
        n200 = Unbundle By Name(w434) -> ("status"=w447:bool)
        n201 = Unbundle By Name(w432) -> ("status"=w446:bool)
        n202 = Unbundle By Name(w430) -> ("status"=w442:bool)
        n203 = Or(x=w449, y=w448) -> (x .or. y?=w444:bool)
        n204 = Or(x=w447, y=w446) -> (x .or. y?=w445:bool)
        n205 = Or(x=w442, y="stop") -> (x .or. y?=w441:bool)
        n206 = Or(x=w445, y=w441) -> (x .or. y?=w443:bool)
        n207 = Or(x=w444, y=w443) -> (x .or. y?=w439:bool)
      }
      n208 = VISA Close(VISA resource name=w393, error in (no error)=w394) -> (error out=w397:errorcluster)
      n209 = VISA Close(VISA resource name=w398, error in (no error)=w404) -> (error out=w405:errorcluster)
      n210 = VISA Close(VISA resource name=w392, error in (no error)=w391) -> (error out=w396:errorcluster)
      n211 = VISA Close(VISA resource name=w389, error in (no error)=w390) -> (error out=w395:errorcluster)
      n212 = VISA Close(VISA resource name=w413, error in (no error)=w414) -> (error out=w412:errorcluster)
      n213 = call <vilib>:"Simple Error Handler.vi"("error in (no error)"=w397) -> ()  [unwired: 1 in, 8 out]
      n214 = call <vilib>:"Simple Error Handler.vi"("error in (no error)"=w405) -> ()  [unwired: 1 in, 8 out]
      n215 = call <vilib>:"Simple Error Handler.vi"("error in (no error)"=w396) -> ()  [unwired: 1 in, 8 out]
      n216 = call <vilib>:"Simple Error Handler.vi"("error in (no error)"=w395) -> ()  [unwired: 1 in, 8 out]
      n217 = call <vilib>:"Simple Error Handler.vi"("error in (no error)"=w412) -> ()  [unwired: 1 in, 8 out]
    }
  }
  n218 = while {
    stop <- w567 continue-if-true
    n219 = case shown="False" "RECORD" {
      selector: "RECORD" -> [w570 _]
      tunnel: [w569 w571] -> w567
      frame False {
        n220 = Not(x=w570) -> (.not. x?=w569:bool)
      }
      frame True {
        w593 = 10214 items=["High"=10192, "Low"=10214] ("Idle State")
        w594 = 10280 items=["Rising"=10280, "Falling"=10171] ("edge")
        w620 = 10123 items=["Finite Samples"=10178, "Continuous Samples"=10123, "Hardware Timed Single Point"=12522] ("sample mode")
        w632 = u16 0 items=["unsigned binary", "offset binary", "2's complement"] ("data format (offset binary)")
        w639 = 0 items=["one channel for each line", "one channel for all lines"] ("line grouping")
        w640 = 10123 items=["Finite Samples"=10178, "Continuous Samples"=10123, "Hardware Timed Single Point"=12522] ("sample mode")
        w643 = T2 3 items=["no dialog", "OK message", "continue or stop message", "OK message + warnings", "continue/stop + warnings"] ("type of dialog (OK msg:1)")
        w647 = T2 3 items=["no dialog", "OK message", "continue or stop message", "OK message + warnings", "continue/stop + warnings"] ("type of dialog (OK msg:1)")
        n221 = call-poly <vilib>:"DAQmx Create Virtual Channel.vi"("maximum value"="Maximum Value", "minimum value"="Minimum Value", "physical channels"="Physical Channel") -> ("task out"=w622:refnum<k21>, "error out"=w621:errorcluster)  [unwired: 11 in]
        n222 = call-poly <vilib>:"DAQmx Create Virtual Channel.vi"("lines"="Digital Output (Camera Trigger)", "line grouping"=w639) -> ("task out"=w642:refnum<k21>, "error out"=w641:errorcluster)  [unwired: 12 in]
        n223 = call <vilib>:"Square Waveform.vi"("duty cycle (%)"="duty cycle (%)", "sampling info"="sampling info", "phase"="phase", "amplitude"="amplitude", "frequency"="frequency") -> ("signal out"=w638:waveform(dbl))  [unwired: 5 in, 1 out]
        n224 = call-poly <vilib>:"DAQmx Timing.vi"("task/channels in"=w622, "sample mode"=w620, "rate"="Sample Clock Rate", "error in"=w621) -> ("task out"=w599:refnum<k21>, "error out"=w598:errorcluster)  [unwired: 10 in]
        n225 = call-poly <vilib>:"DAQmx Timing.vi"("task/channels in"=w642, "sample mode"=w640, "rate"="Sample Clock Rate", "source"=tag "/Dev1/ao/SampleClock", "error in"=w641) -> ("task out"=w602:refnum<k21>, "error out"=w601:errorcluster)  [unwired: 9 in]
        n226 = Divide(x="amplitude", y=2.0) -> (x/y=w606:dbl)
        n227 = call "Get Terminal Name with Device Prefix.vi"("error in (no error)"=w601, "Local Terminal Name"="Ctr0InternalOutput" ("terminal"), "task/channels in"=w602) -> ("error out"=w587:errorcluster, "Terminal Name with Device Prefix"=w600:tag, "task out"=w588:refnum<k21>)  [unwired: 1 in, 5 out]
        n228 = call-poly <vilib>:"Analog to Digital.vi"("data format (offset binary)"=w632, "resolution (16 bit)"=1, "analog waveform"=w638) -> ("digital waveform"=w626:digitalwaveform)  [unwired: 5 in, 3 out]
        n229 = call-poly <vilib>:"DAQmx Trigger.vi"("task/channels in"=w599, "source"=w600, "edge"=w594, "error in"=w598) -> ("task out"=w597:refnum<k21>, "error out"=w596:errorcluster)  [unwired: 1 in, 9 out]
        n230 = call <vilib>:"Square Waveform.vi"("duty cycle (%)"="duty cycle (%)", "offset"=w606, "sampling info"="sampling info", "phase"="phase", "amplitude"=w606, "frequency"="frequency") -> ("signal out"=w616:waveform(dbl))  [unwired: 4 in, 1 out]
        n231 = Build Array(w626, w626) -> (w631:digitalwaveform[])
        n232 = call-poly <vilib>:"DAQmx Write.vi"("task/channels in"=w597, "data"=w616, "error in"=w596) -> ("task out"=w613:refnum<k21>, "error out"=w612:errorcluster)  [unwired: 10 in, 1 out]
        n233 = call-poly <vilib>:"DAQmx Write.vi"("task/channels in"=w588, "data"=w631, "error in"=w587) -> ("task out"=w595:refnum<k21>, "error out"=w585:errorcluster)  [unwired: 10 in, 1 out]
        n234 = call <vilib>:"DAQmx Start Task.vi"("task/channels in"=w613, "error in"=w612) -> ("task out"=w611:refnum<k21>, "error out"=w586:errorcluster)  [unwired: 12 in]
        n235 = call-poly <vilib>:"DAQmx Create Virtual Channel.vi"("high time"=1.0 ("High Time"), "low time"=0.5 ("Low Time"), "counter"=tag "Dev1/ctr0" ("Counter(s)"), "idle state"=w593, "initial delay"=0.0 ("Initial Delay")) -> ("task out"=w581:refnum<k21>, "error out"=w582:errorcluster)  [unwired: 4 in, 5 out]
        n236 = Merge Errors(w585, w586) -> (w584:errorcluster)
        n237 = call <vilib>:"DAQmx Start Task.vi"("task/channels in"=w595, "error in"=w584) -> ("task out"=w645:refnum<k21>, "error out"=w583:errorcluster)  [unwired: 12 in]
        n238 = Merge Errors(w582, w583) -> (w580:errorcluster)
        n239 = call-poly <vilib>:"DAQmx Create Virtual Channel.vi"("maximum value"="Maximum Value", "minimum value"="Minimum Value", "physical channels"="Physical Channel") -> ("task out"=w630:refnum<k21>, "error out"=w629:errorcluster)  [unwired: 11 in]
        n240 = call <vilib>:"DAQmx Start Task.vi"("task/channels in"=w581, "error in"=w580) -> ("task out"=w578:refnum<k21>, "error out"=w579:errorcluster)  [unwired: 12 in]
        n241 = while {
          tunnel: w645 -> [w666]
          tunnel: [w665] -> w625
          tunnel: w579 -> [w664]
          tunnel: w630 -> [w660]
          tunnel: w629 -> [w661]
          tunnel: [w659] -> w627
          tunnel: [w658] -> w628
          tunnel: w611 -> [w656]
          tunnel: [w655] -> w610
          tunnel: [w653] -> w574
          tunnel: [w649] -> w571
          stop <- w649 stop-if-true
          w663 = u32 100  # millisecond multiple
          n242 = call <vilib>:"DAQmx Is Task Done.vi"("task/channels in"=w666, "error in"=w664) -> ("task out"=w665:refnum<k21>, "error out"=w654:errorcluster)  [unwired: 11 in, 1 out]
          n243 = case shown="True" "On / Off" {
            tunnel: w660 -> [w667 w677]
            tunnel: w661 -> [_ w676]
            tunnel: [w669 w672] -> w658
            tunnel: [w668 w673] -> w659
            frame False {
              n244 = call-poly <vilib>:"DAQmx Write.vi"("task/channels in"=w667, "data"=0.0 ("Voltage Output 2"), "timeout"=10.0) -> ("task out"=w668:refnum<k21>, "error out"=w669:errorcluster)  [unwired: 10 in, 1 out]
            }
            frame True {
              n245 = call-poly <vilib>:"DAQmx Write.vi"("task/channels in"=w677, "data"="Voltage Output", "timeout"=10.0, "error in"=w676) -> ("task out"=w673:refnum<k21>, "error out"=w672:errorcluster)  [unwired: 9 in, 1 out]
            }
          }
          n246 = Wait Until Next ms Multiple(millisecond multiple=w663) -> ()  [unwired: 1 out]
          n247 = call <vilib>:"DAQmx Is Task Done.vi"("task/channels in"=w656, "error in"=w654) -> ("task out"=w655:refnum<k21>, "error out"=w653:errorcluster)  [unwired: 11 in, 1 out]
          n248 = Unbundle By Name(w653) -> ("status"=w650:bool)
          n249 = Unbundle By Name(w658) -> ("status"=w651:bool)
          n250 = Or(x=w650, y=w651) -> (x .or. y?=w652:bool)
          n251 = Or(x="STOP", y=w652) -> (x .or. y?=w649:bool)
        }
        n252 = call <vilib>:"DAQmx Clear Task.vi"("task in"=w627, "error in"=w628) -> ("error out"=w646:errorcluster)  [unwired: 13 in]
        n253 = call <vilib>:"Simple Error Handler.vi"("type of dialog (OK msg:1)"=w647, "error in (no error)"=w646) -> ()  [unwired: 3 in, 5 out]
        n254 = call-poly <vilib>:"DAQmx Write.vi"("task/channels in"=w625, "data"=bool[] [], "error in"=w574) -> ("task out"=w624:refnum<k21>, "error out"=w573:errorcluster)  [unwired: 10 in, 1 out]
        n255 = call <vilib>:"DAQmx Clear Task.vi"("task in"=w610, "error in"=w573) -> ("error out"=w572:errorcluster)  [unwired: 13 in]
        n256 = call <vilib>:"DAQmx Clear Task.vi"("task in"=w624, "error in"=w572) -> ("error out"=w577:errorcluster)  [unwired: 13 in]
        n257 = call <vilib>:"DAQmx Clear Task.vi"("task in"=w578, "error in"=w577) -> ("error out"=w576:errorcluster)  [unwired: 13 in]
        n258 = call <vilib>:"Simple Error Handler.vi"("type of dialog (OK msg:1)"=w643, "error in (no error)"=w576) -> ()  [unwired: 3 in, 5 out]
      }
    }
  }
